vi "Set startup speed.vi"(8 "error in (no error)":errorcluster, 11 "StageSPIM in":refnum<class "StageSPIM.lvclass">) -> (0 "error out":errorcluster, 3 "StageSPIM out":refnum<class "StageSPIM.lvclass">)   [LabVIEW 2012, in "StageSPIM.lvclass"]
uses:
  StageSPIM.lvclass
  StageSPIM.lvclass/StageSPIM.ctl
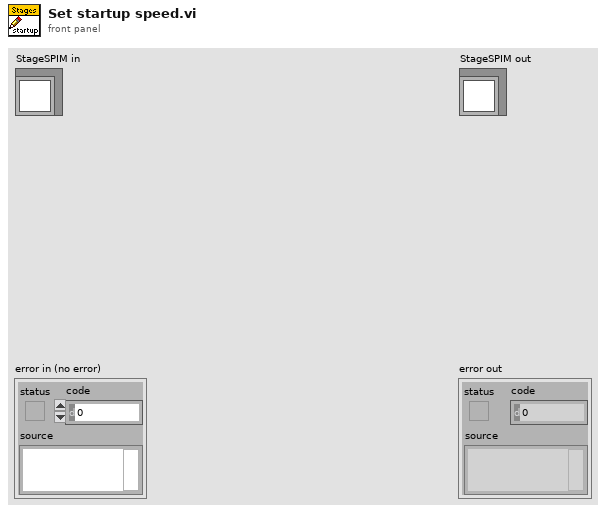
[diagram p1: front panel]
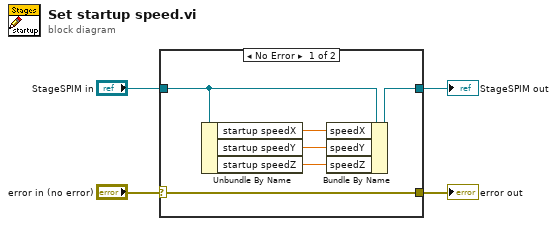
[diagram p0: block diagram]
diagram:
  n1 = case shown="No Error" "error in (no error)" {
    selector: "error in (no error)" -> [w10 w12]
    tunnel: [w10 w12] -> w3
    tunnel: [w8 w11] -> w1
    tunnel: "StageSPIM in" -> [w9 w11]
    frame No Error {
      n2 = Unbundle By Name(w9) -> ("startup speedX"=w7:dbl[unit], "startup speedY"=w6:dbl[unit], "startup speedZ"=w5:dbl[unit])
      n3 = Bundle By Name(cluster=w9, "speedX"=w7, "speedY"=w6, "speedZ"=w5) -> (w8:refnum<class "StageSPIM.lvclass">)
    }
    frame Error {
    }
  }
  "error out" <- w3
  "StageSPIM out" <- w1
